vi "Change Settings.vi"(8 "error in (no error)":errorcluster) -> (0 "error out":errorcluster)   [LabVIEW 2020, in "MacroAssert.lvlib"]
doc: "Displays a window to change any settings that have been established in the application."
uses:
  MacroAssert.lvlib
  CTLs/Hotkey Type.ctl
  CTLs/Hotkey Values.ctl
  CTLs/FGV Actions.ctl
  2b057859-5186-41e9-9ab4-790756e7a186.vi
  a5ac09e5-38d3-43bc-9feb-68748838b8f7.vi
  <vilib>/Utility/inputDevices.llb/closeKeyboard.vi
  <vilib>/Utility/inputDevices.llb/keyboardAcquire.vi
  FaKI State Machine/FaKI State Machine.lvlib
panel:
  in  "Hotkey Type":T1
  in  "Start/Stop":bool
  in  "Exit":bool
  # "Change Hotkey\nPress Start Listening and hold down a key combination for five seconds to assign it as a hotkey."
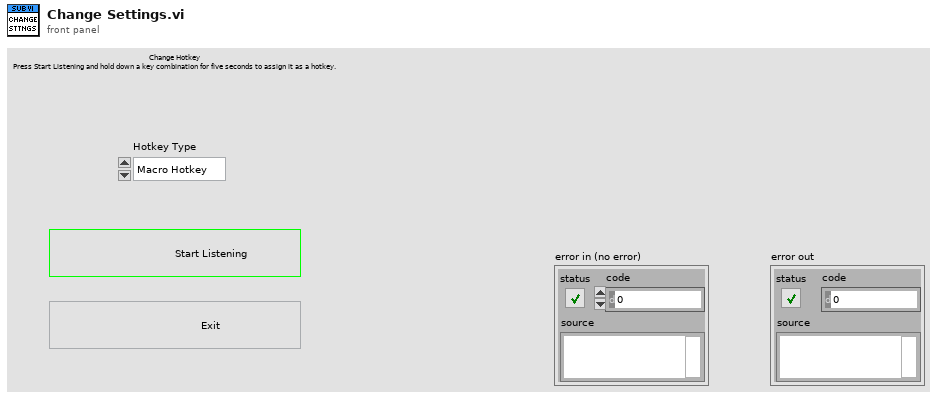
[diagram p1: front panel]
types:
  T1 = typedef "MacroAssert.lvlib/Hotkey Type.ctl" = enum16{"Macro Hotkey", "Abort Hotkey"}
  T2 = enum32{"Invalid", "Standard", "Closed", "Hidden", "Minimized", "Maximized"}
  T3 = enum32{"invalid app kind", "Development System", "Run Time System", "Student Edition", "Embedded LabVIEW", "Evaluation", "Custom"}
  T4 = typedef "MacroAssert.lvlib/FGV Actions.ctl" = enum16{"Read", "Write"}
  T5 = typedef "MacroAssert.lvlib/Hotkey Values.ctl" = cluster{"Macro Hotkey":enum16{"0", "1", "2", "3", "4", "5", "6", "7", "8", "9", "A", "B", "C", "D", "E", "F", "G", "H", "I", "J", "K", "L", "M", "N", "O", "P", "Q", "R", "S", "T", "U", "V", "W", "X", "Y", "Z", "F1", "F2", "F3", "F4", "F5", "F6", "F7", "F8", "F9", "F10", "F11", "F12", "F13", "F14", "F15", "ADD", "BACK", "BACKSLASH", "CAPITAL", "COMMA", "DECIMAL", "DELETE", "DIVIDE", "DOWN", "END", "EQUALS", "ESCAPE", "GRAVE (`)", "HOME", "INSERT", "LBRACKET", "LCONTROL", "LEFT", "L ALT", "LSHIFT", "LWIN", "MINUS", "MULTIPLY", "NEXT", "NUMLOCK", "NUMPAD_0", "NUMPAD_1", "NUMPAD_2", "NUMPAD_3", "NUMPAD_4", "NUMPAD_5", "NUMPAD_6", "NUMPAD_7", "NUMPAD_8", "NUMPAD_9", "PAUSE", "PERIOD", "PRIOR (PG UP)", "RBRACKET", "RCONTROL", "RETURN", "RIGHT", "R ALT", "RSHIFT", "RWIN", "SCROLL", "SEMICOLON", "SLASH", "SPACE", "SUBTRACT", "TAB", "UP", "ENTER (num pad)", "' (quote)"}[], "Abort Hotkey":enum16{"0", "1", "2", "3", "4", "5", "6", "7", "8", "9", "A", "B", "C", "D", "E", "F", "G", "H", "I", "J", "K", "L", "M", "N", "O", "P", "Q", "R", "S", "T", "U", "V", "W", "X", "Y", "Z", "F1", "F2", "F3", "F4", "F5", "F6", "F7", "F8", "F9", "F10", "F11", "F12", "F13", "F14", "F15", "ADD", "BACK", "BACKSLASH", "CAPITAL", "COMMA", "DECIMAL", "DELETE", "DIVIDE", "DOWN", "END", "EQUALS", "ESCAPE", "GRAVE (`)", "HOME", "INSERT", "LBRACKET", "LCONTROL", "LEFT", "L ALT", "LSHIFT", "LWIN", "MINUS", "MULTIPLY", "NEXT", "NUMLOCK", "NUMPAD_0", "NUMPAD_1", "NUMPAD_2", "NUMPAD_3", "NUMPAD_4", "NUMPAD_5", "NUMPAD_6", "NUMPAD_7", "NUMPAD_8", "NUMPAD_9", "PAUSE", "PERIOD", "PRIOR (PG UP)", "RBRACKET", "RCONTROL", "RETURN", "RIGHT", "R ALT", "RSHIFT", "RWIN", "SCROLL", "SEMICOLON", "SLASH", "SPACE", "SUBTRACT", "TAB", "UP", "ENTER (num pad)", "' (quote)"}[]}
  T6 = cluster{"Core":cluster{"Current VI Reference":refnum<vi>, "Close Panel on Exit?":bool}, "Keyboard":refnum<k1>, "Last":enum16{"0", "1", "2", "3", "4", "5", "6", "7", "8", "9", "A", "B", "C", "D", "E", "F", "G", "H", "I", "J", "K", "L", "M", "N", "O", "P", "Q", "R", "S", "T", "U", "V", "W", "X", "Y", "Z", "F1", "F2", "F3", "F4", "F5", "F6", "F7", "F8", "F9", "F10", "F11", "F12", "F13", "F14", "F15", "ADD", "BACK", "BACKSLASH", "CAPITAL", "COMMA", "DECIMAL", "DELETE", "DIVIDE", "DOWN", "END", "EQUALS", "ESCAPE", "GRAVE (`)", "HOME", "INSERT", "LBRACKET", "LCONTROL", "LEFT", "L ALT", "LSHIFT", "LWIN", "MINUS", "MULTIPLY", "NEXT", "NUMLOCK", "NUMPAD_0", "NUMPAD_1", "NUMPAD_2", "NUMPAD_3", "NUMPAD_4", "NUMPAD_5", "NUMPAD_6", "NUMPAD_7", "NUMPAD_8", "NUMPAD_9", "PAUSE", "PERIOD", "PRIOR (PG UP)", "RBRACKET", "RCONTROL", "RETURN", "RIGHT", "R ALT", "RSHIFT", "RWIN", "SCROLL", "SEMICOLON", "SLASH", "SPACE", "SUBTRACT", "TAB", "UP", "ENTER (num pad)", "' (quote)"}[], "Hotkeys":T5}
  T7 = enum16{"0", "1", "2", "3", "4", "5", "6", "7", "8", "9", "A", "B", "C", "D", "E", "F", "G", "H", "I", "J", "K", "L", "M", "N", "O", "P", "Q", "R", "S", "T", "U", "V", "W", "X", "Y", "Z", "F1", "F2", "F3", "F4", "F5", "F6", "F7", "F8", "F9", "F10", "F11", "F12", "F13", "F14", "F15", "ADD", "BACK", "BACKSLASH", "CAPITAL", "COMMA", "DECIMAL", "DELETE", "DIVIDE", "DOWN", "END", "EQUALS", "ESCAPE", "GRAVE (`)", "HOME", "INSERT", "LBRACKET", "LCONTROL", "LEFT", "L ALT", "LSHIFT", "LWIN", "MINUS", "MULTIPLY", "NEXT", "NUMLOCK", "NUMPAD_0", "NUMPAD_1", "NUMPAD_2", "NUMPAD_3", "NUMPAD_4", "NUMPAD_5", "NUMPAD_6", "NUMPAD_7", "NUMPAD_8", "NUMPAD_9", "PAUSE", "PERIOD", "PRIOR (PG UP)", "RBRACKET", "RCONTROL", "RETURN", "RIGHT", "R ALT", "RSHIFT", "RWIN", "SCROLL", "SEMICOLON", "SLASH", "SPACE", "SUBTRACT", "TAB", "UP", "ENTER (num pad)", "' (quote)"}[]
  T8 = cluster{"Current VI Reference":refnum<vi>, "Close Panel on Exit?":bool}
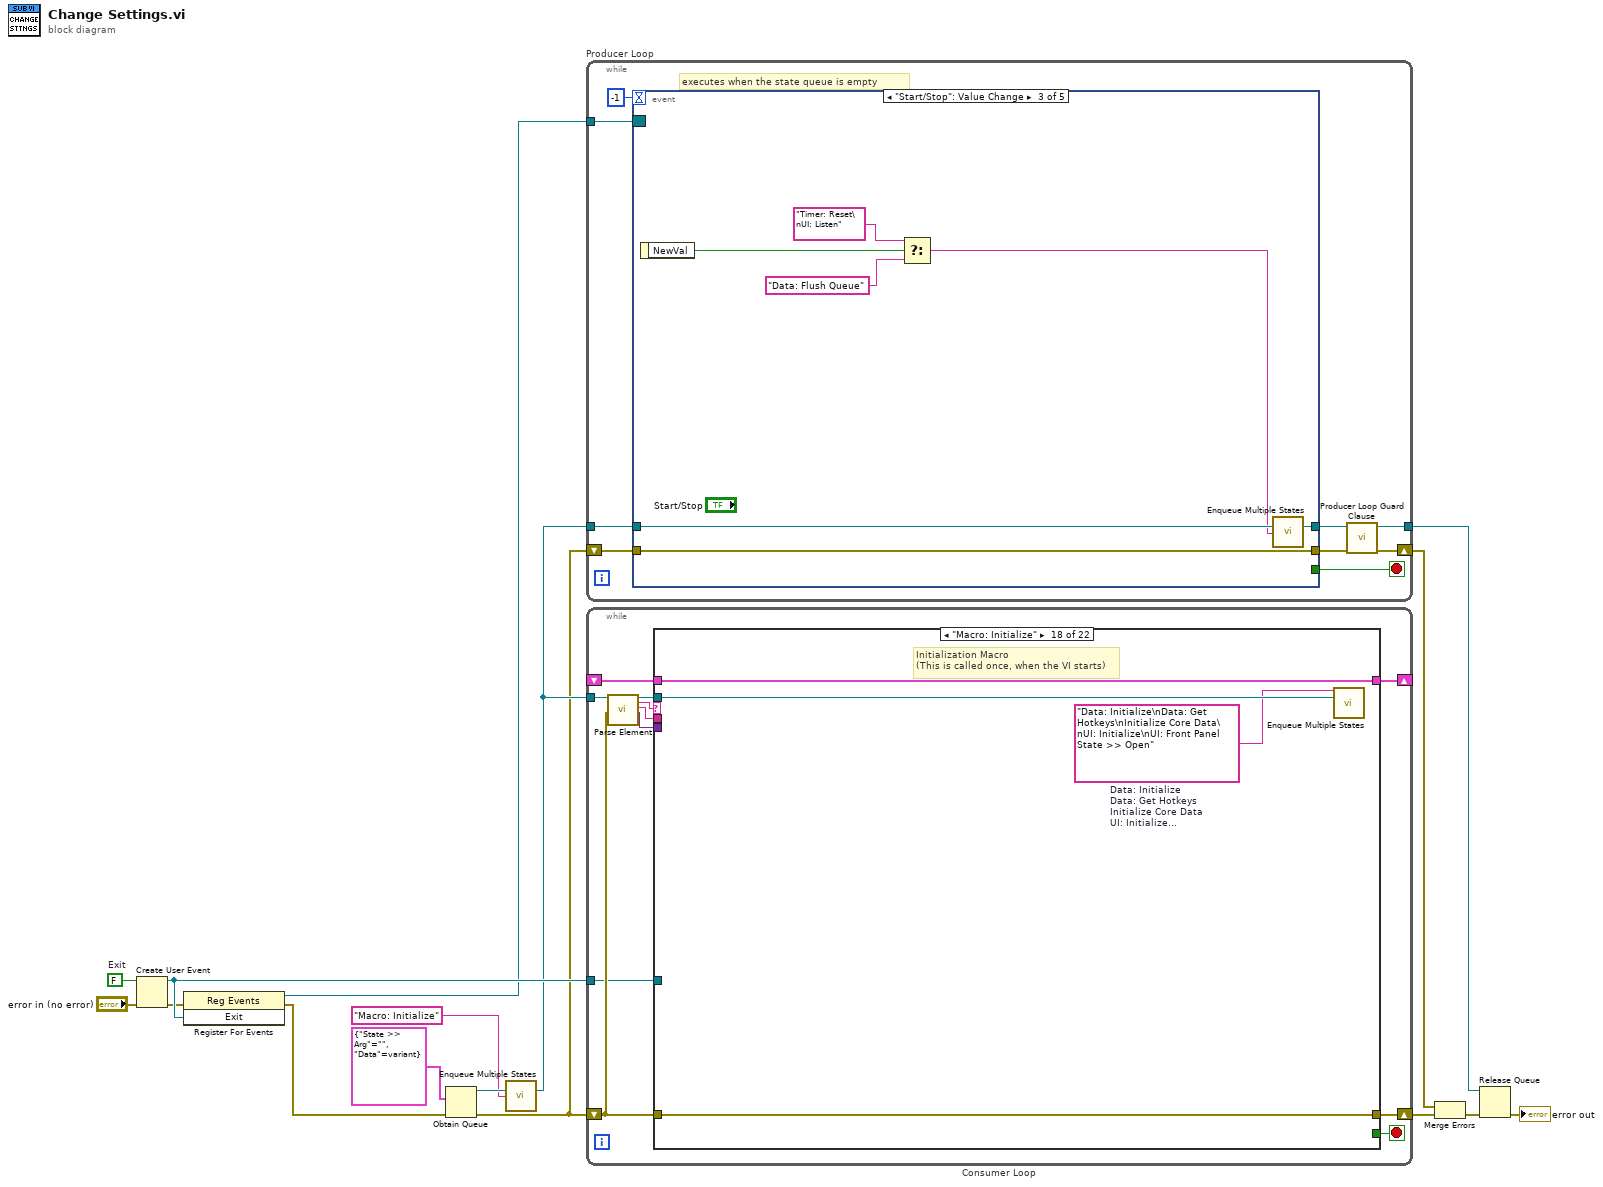
[diagram p0: block diagram]
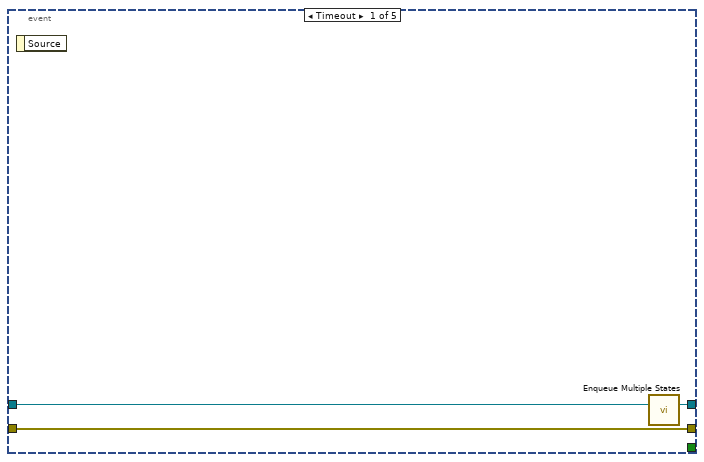
[diagram p2: hidden frame]
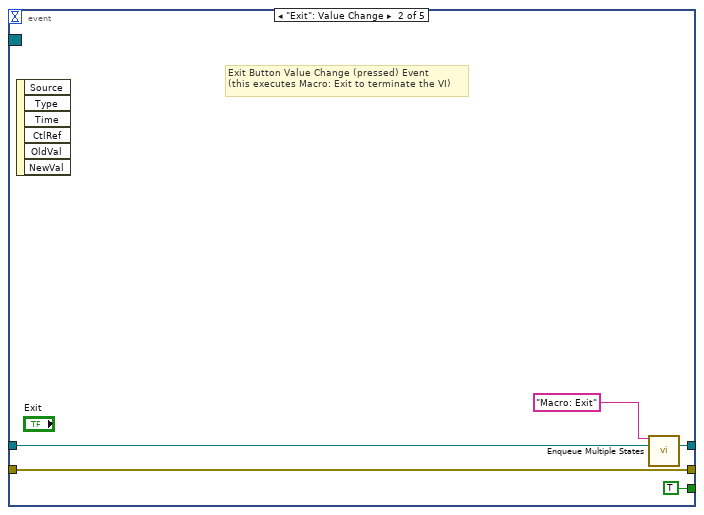
[diagram p3: hidden frame]
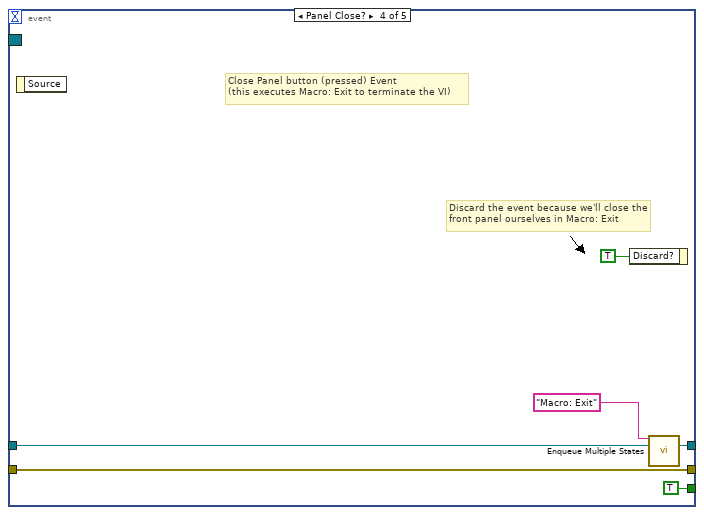
[diagram p4: hidden frame]
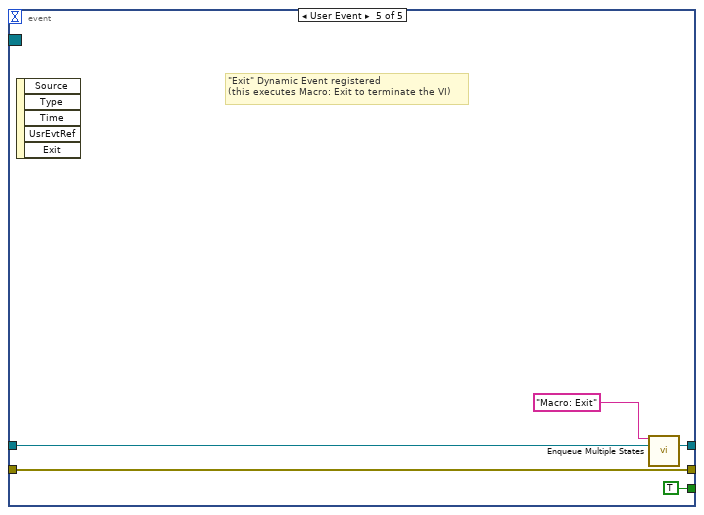
[diagram p5: hidden frame]
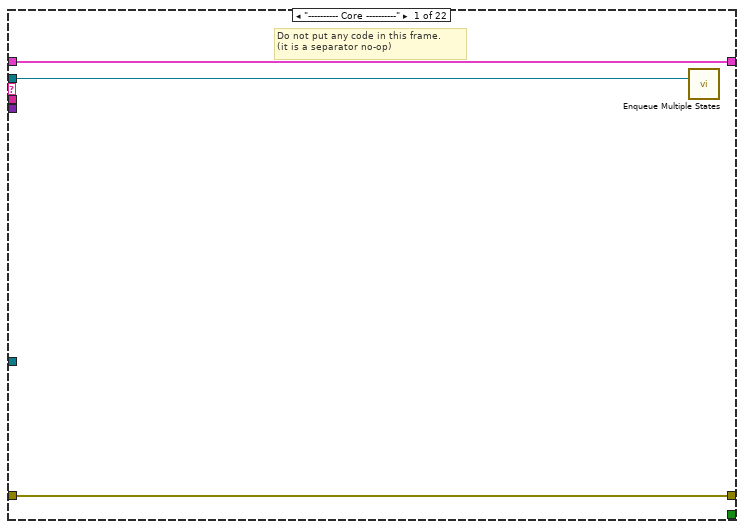
[diagram p6: hidden frame]
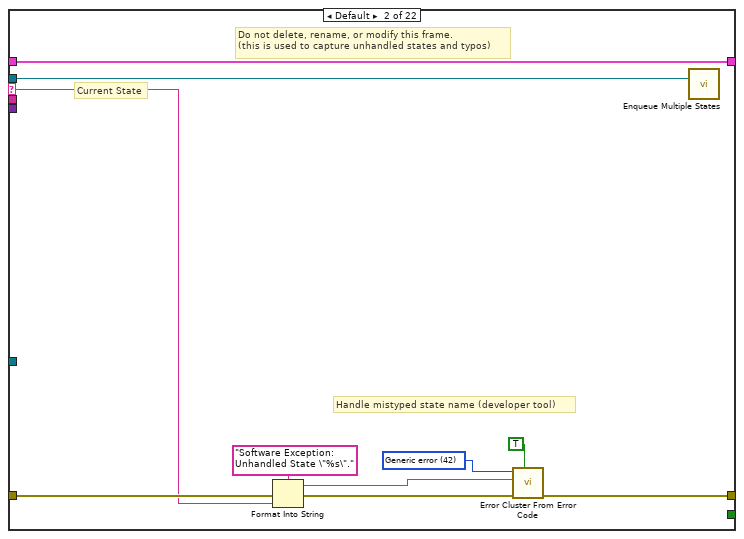
[diagram p7: hidden frame]
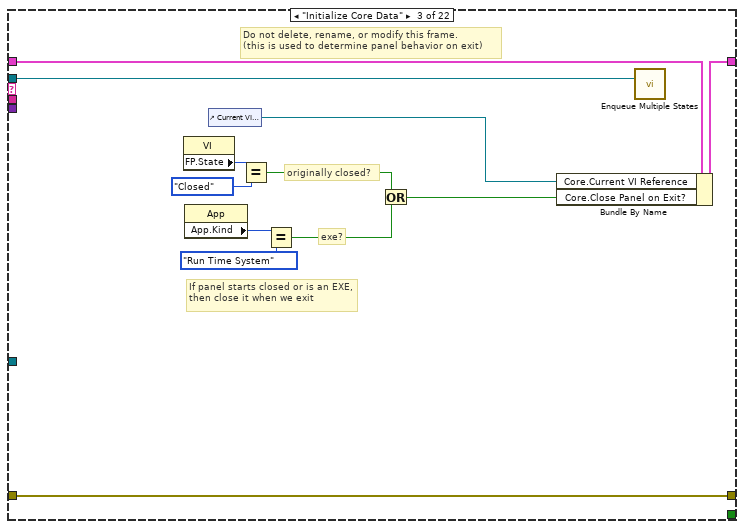
[diagram p8: hidden frame]
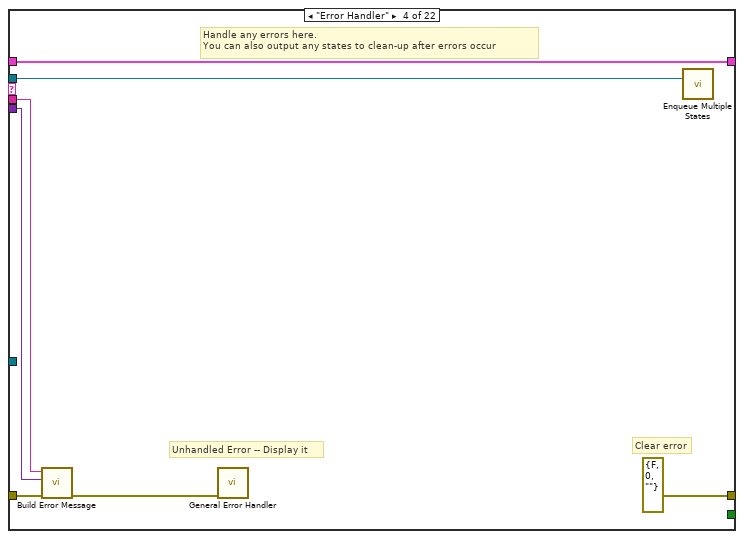
[diagram p9: hidden frame]
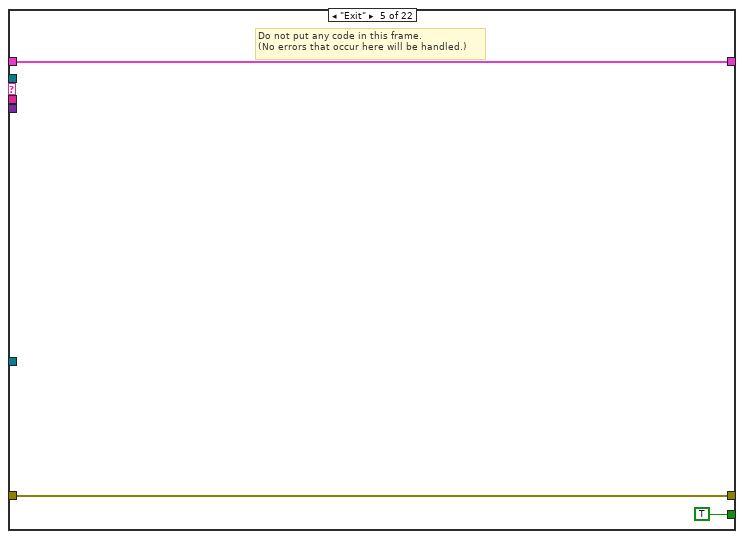
[diagram p10: hidden frame]
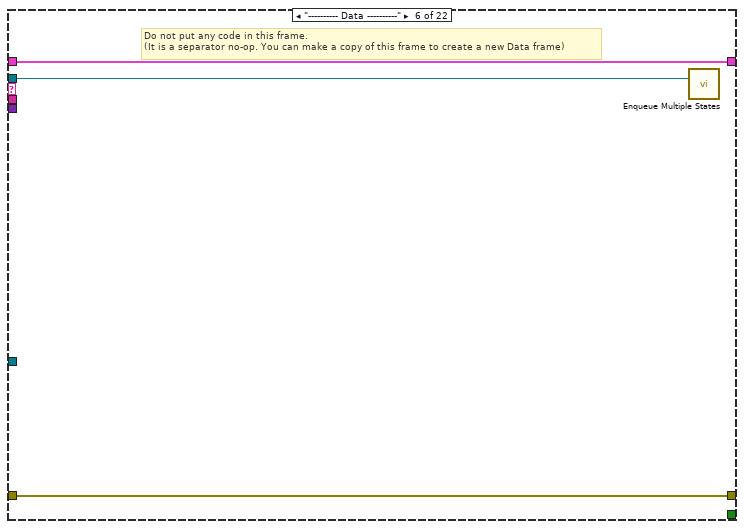
[diagram p11: hidden frame]
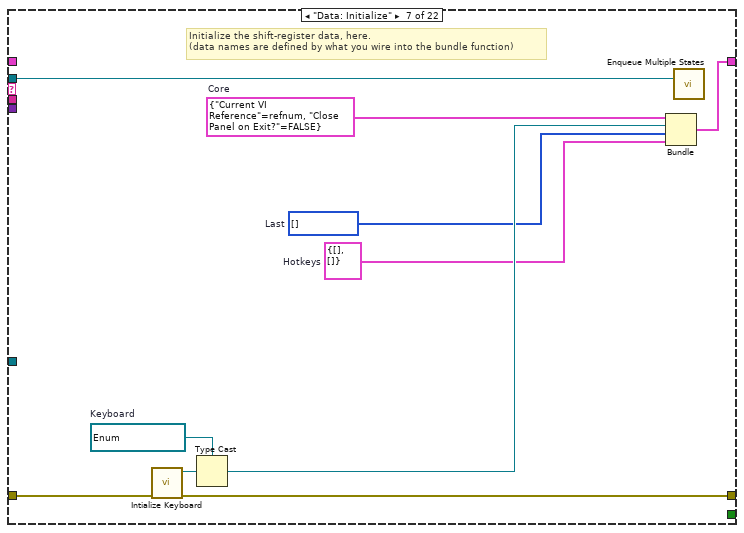
[diagram p12: hidden frame]
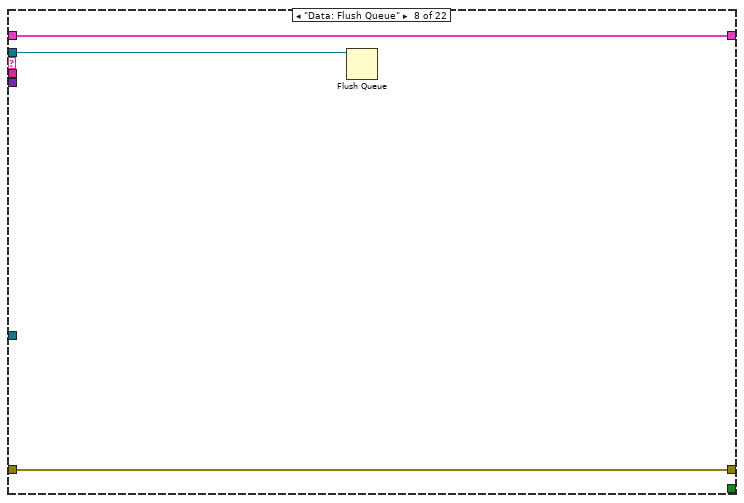
[diagram p13: hidden frame]
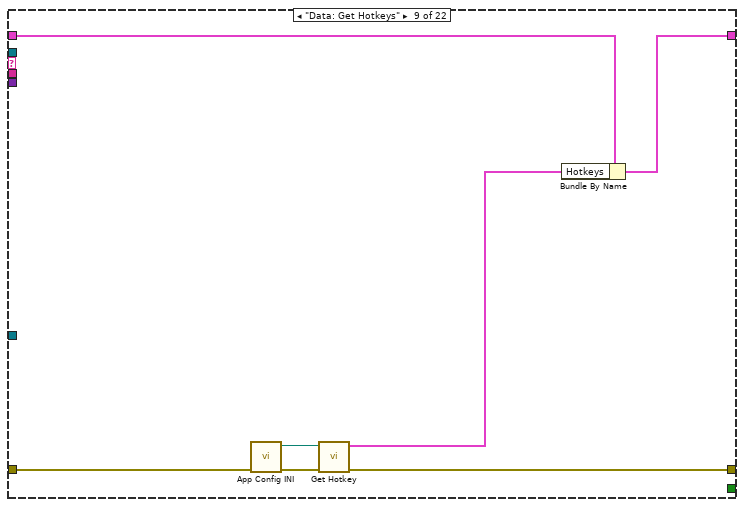
[diagram p14: hidden frame]
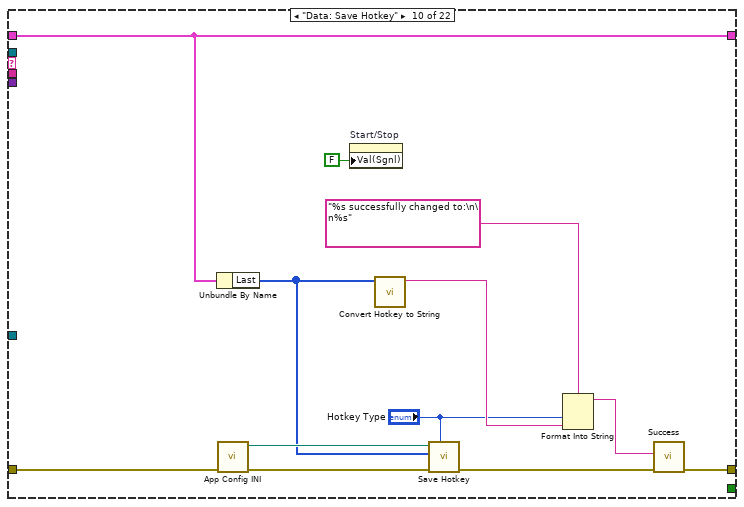
[diagram p15: hidden frame]
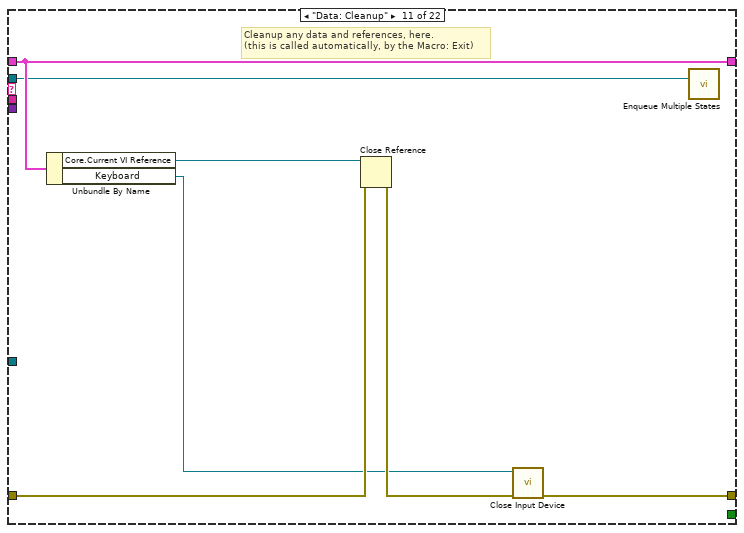
[diagram p16: hidden frame]
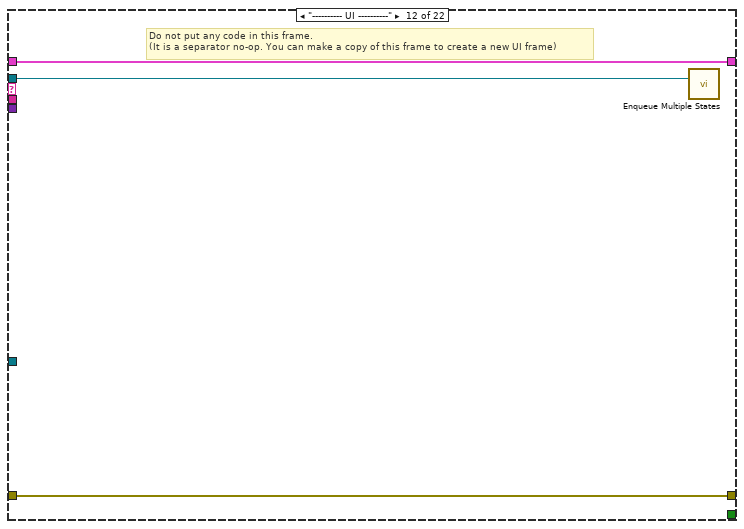
[diagram p17: hidden frame]
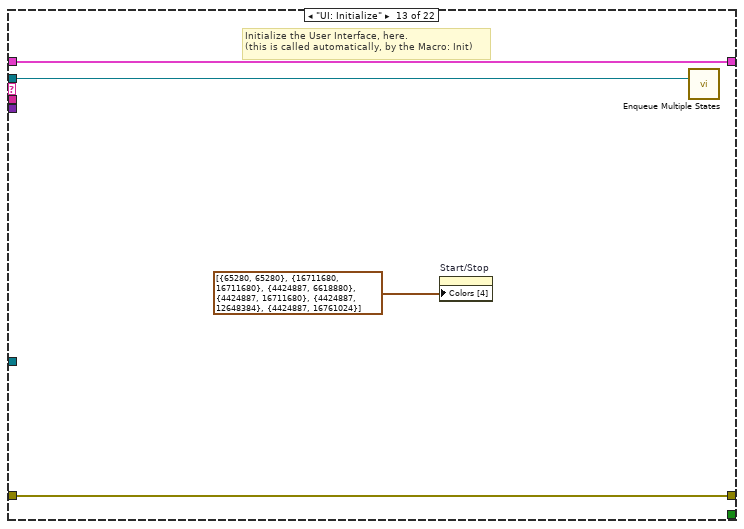
[diagram p18: hidden frame]
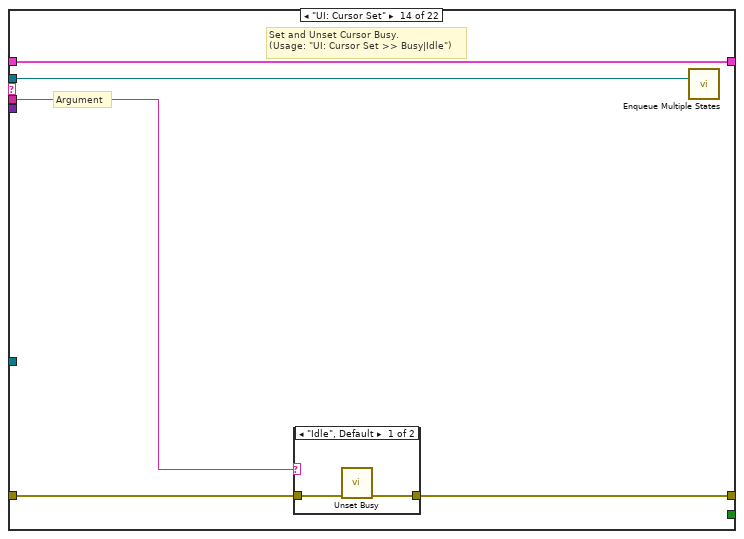
[diagram p19: hidden frame]
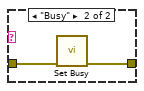
[diagram p20: hidden frame]
diagram:
  w13 = FALSE  # Exit
  n1 = Create User Event(user event datatype=w13, error in="error in (no error)") -> (user event=w16:refnum<user-event>, error out=w12:errorcluster)
  n2 = register-events(error in=w12, w16) -> (reference out=w15:refnum<event-registration>, error out=w14:errorcluster)  [unwired: 1 in]
  n3 = Obtain Queue(element data type=cluster{"State >> Arg":string, "Data":variant} {"State >> Arg"="", "Data"=variant}, error in (no error)=w14) -> (queue out=w6:refnum<queue>, error out=w3:errorcluster)  [unwired: 3 in, 1 out]
  n4 = call "Enqueue Multiple States.vi"("queue in"=w6, "State(s) at Back"="Macro: Initialize") -> ("queue out"=w7:refnum<queue>)  [unwired: 13 in]
  n5 = while "Producer Loop" {
    shift-right: [w20] -> w9
    shift-left: w3 -> [w25]
    tunnel: w15 -> [w17]
    tunnel: w7 -> [w23]
    tunnel: [w18] -> w11
    stop <- w22 stop-if-true
    # "executes when the state queue is empty"
    n6 = event shown="[2] \"Start/Stop\": Value Change" {
      selector: w17 -> [_ _ _ _ _]
      dyn-events: _ -> [_ _ _ _ _]
      timeout: -1 ("Timeout") -> [_ _ _ _ _]
      tunnel: [w26 w33 w40 w46 w51] -> w21
      tunnel: w25 -> [w26 w33 w40 w46 w51]
      tunnel: w23 -> [w27 w32 w39 w43 w49]
      tunnel: [w28 w30 w38 w42 w48] -> w19
      tunnel: [_ TRUE _ TRUE TRUE] -> w22
      event Timeout {
        n7 = event-data() -> ()  [unwired: 1 in, 1 out]
        n8 = call "Enqueue Multiple States.vi"("queue in"=w27) -> ("queue out"=w28:refnum<queue>)  [unwired: 14 in]
      }
      event "Exit": Value Change {
        # "Exit Button Value Change (pressed) Event\n(this executes Macro: Exit to terminate the VI)"
        n9 = event-data() -> ()  [unwired: 1 in, 6 out]
        n10 = call "Enqueue Multiple States.vi"("State(s) at Front"="Macro: Exit", "queue in"=w32) -> ("queue out"=w30:refnum<queue>)  [unwired: 13 in]
      }
      event "Start/Stop": Value Change {
        n11 = event-data() -> ("NewVal"=w37:bool)  [unwired: 1 in]
        n12 = Select(t="Timer: Reset\nUI: Listen", s=w37, f="Data: Flush Queue") -> (s? t:f=w34:string)
        n13 = call "Enqueue Multiple States.vi"("queue in"=w39, "State(s) at Back"=w34) -> ("queue out"=w38:refnum<queue>)  [unwired: 13 in]
      }
      event Panel Close? {
        # "Discard the event because we'll close the front panel ourselves in Macro: Exit"
        # "Close Panel button (pressed) Event\n(this executes Macro: Exit to terminate the VI)"
        n14 = event-data() -> ()  [unwired: 1 in, 1 out]
        n15 = event-data("Discard?"=TRUE) -> ()  [unwired: 1 in, 1 out]
        n16 = call "Enqueue Multiple States.vi"("State(s) at Front"="Macro: Exit", "queue in"=w43) -> ("queue out"=w42:refnum<queue>)  [unwired: 13 in]
      }
      event User Event {
        # "\"Exit\" Dynamic Event registered\n(this executes Macro: Exit to terminate the VI)"
        n17 = event-data() -> ()  [unwired: 1 in, 5 out]
        n18 = call "Enqueue Multiple States.vi"("State(s) at Front"="Macro: Exit", "queue in"=w49) -> ("queue out"=w48:refnum<queue>)  [unwired: 13 in]
      }
    }
    n19 = call "Producer Loop Guard Clause.vi"("error in (no error)"=w21, "queue in"=w19) -> ("error out"=w20:errorcluster, "queue out"=w18:refnum<queue>)  [unwired: 8 in]
  }
  n20 = while "Consumer Loop" {
    shift-right: [w59] -> _
    shift-left: _ -> [w58]
    shift-right: [w62] -> w8
    shift-left: w3 -> [w61]
    tunnel: w7 -> [w57]
    tunnel: w16 -> [w52]
    stop <- w60 stop-if-true
    n21 = call "Parse Element.vi"("queue in"=w57, "error in (no error)"=w61) -> ("queue out"=w56:refnum<queue>, "State"=w55:string, "Arg"=w54:string, "Data"=w53:variant)  [unwired: 14 in]
    n22 = case shown="\"Macro: Initialize\"" w55 {
      selector: w55 -> [_ w67 _ _ _ _ _ _ _ _ _ _ _ _ _ _ _ _ _ _ _ _]
      tunnel: w56 -> [w63 w66 w76 w92 _ w98 w108 w113 _ _ w136 w140 w144 w147 w156 w239 w262 w266 w272 w278 _ w287]
      tunnel: w54 -> [_ _ _ w88 _ _ _ _ _ _ _ _ _ w148 w157 _ _ _ _ _ _ _]
      tunnel: w58 -> [w64 w69 w82 w93 w96 w99 _ w112 w119 w125 w137 w141 w145 w149 w159 w238 w263 w267 w276 w279 w285 w294]
      tunnel: [w65 w74 w87 errorcluster {"status"=FALSE, "code"=0, "source"=""} ("error out") w97 w100 w103 w111 w117 w130 w134 w142 w146 w150 w160 w247 w264 w268 w277 w280 w283 w292] -> w62
      tunnel: w61 -> [w65 w73 w87 w91 w97 w100 w105 w111 w120 w128 w139 w142 w146 w151 w161 w248 w264 w268 w277 w280 w284 w293]
      tunnel: [_ _ _ _ TRUE _ _ _ _ _ _ _ _ _ _ _ _ _ _ _ _ _] -> w60
      tunnel: [w64 w69 w86 w93 w96 w99 w110 w112 w118 w125 w137 w141 w145 w149 w159 w237 w263 w267 w276 w279 w285 w294] -> w59
      tunnel: w53 -> [_ _ _ w89 _ _ _ _ _ _ _ _ _ _ _ _ _ _ _ _ _ _]
      tunnel: w52 -> [_ _ _ _ _ _ _ _ _ _ _ _ _ _ _ _ _ _ _ _ _ _]
      frame "---------- Core ----------" {
        # "Do not put any code in this frame.\n(it is a separator no-op)"
        n23 = call "Enqueue Multiple States.vi"("queue in"=w63) -> ()  [unwired: 14 in, 1 out]
      }
      frame Default {
        w71 = 42 items=["No error", "Argument error", "Memory is full", "Out of zone", "End of file", "File already open", "Generic file I/O error", "File not found", "File permission error", "Disk is full", "Duplicate path", "Too many files open", "System feature not enabled", "Resource file not found", "Cannot add resource", "Resource not found", "Image not found", "Image memory error", "Pen does not exist", "Config type invalid", "Config token not found", "Config parse error", "Config memory error", "Bad external code format", "Bad external code offset", "External code not present", "Null window", "Destroy window error", "Null menu", "Print aborted", "Bad print record", "Print driver error", "Windows error during printing", "Memory error during printing", "Print dialog error", "Generic print error", "Invalid device refnum", "Device not found", "Device parameter error", "Device unit error", "Cannot open device", "Device call aborted", "Generic error", "Cancelled by user", "Object ID too low", "Object ID too high", "Object not in heap", "Unknown heap", "Unknown object (invalid DefProc)", "Unknown object (DefProc not in table)", "Message out of range", "Invalid (null) method", "Unknown message", "Manager call not supported", "Bad address", "Network operation in progress", "Network operation timed out", "Connection is busy", "Network attribute not supported", "Network error", "Address in use", "System out of memory", "Connection aborted", "Connection refused", "Not connected", "Already connected", "Connection closed", "Initialization error (interapplication manager)", "Bad occurrence", "Wait on unbound occurrence handler", "Occurrence queue overflow", "Datalog type conflict", "Unused", "Unrecognized type (interapplication manager)", "Memory corrupt", "Failed to make temporary DLL", "Old CIN version", "Drag socket not found", "Failed to load drop-object", "Failed to register OLE object", "Failed to release OLE object", "Format specifier type mismatch", "Unknown format specifier", "Too few format specifiers", "Too many format specifiers", "Scan failed", "Newer CIN version", "Error converting to variant", "Runtime menu error", "Password tampered", "Variant attribute not found", "Incompatible variant data type", "Event data is not available", "Event Store is not present", "Occurrence is not found", "Event Queue is not created", "Event info is not available", "Refnum passed is NULL", "Error retrieving Class GUID", "Error retrieving CoClass GUID", "Error retrieving TypeLib GUID.", "Bad built application magic bytes.", "Specific driver is different from the specific driver associated with the Logical Name.", "There is no session opened to the class driver.", "Max Error", "MAX - Error with config objects", "MAX - Error loading configuration", "MAX - Group not supported"]
        # "Current State"
        # "Do not delete, rename, or modify this frame.\n(this is used to capture unhandled states and typos)"
        # "Handle mistyped state name (developer tool)"
        n24 = Format Into String(format string="Software Exception: Unhandled State \"%s\"." ("message"), error in=w73, w67) -> (resulting string=w70:string, error out=w75:errorcluster)  [unwired: 1 in]
        n25 = call <vilib>:"Error Cluster From Error Code.vi"("show call chain? (False)"=TRUE, "error in (no error)"=w75, "error message (\"\")"=w70, "error code (0)"=w71) -> ("error out"=w74:errorcluster)  [unwired: 5 in]
        n26 = call "Enqueue Multiple States.vi"("queue in"=w66) -> ()  [unwired: 14 in, 1 out]
      }
      frame "Initialize Core Data" {
        # "Do not delete, rename, or modify this frame.\n(this is used to determine panel behavior on exit)"
        # "originally closed?"
        # "exe?"
        # "If panel starts closed or is an EXE, then close it when we exit"
        n27 = property class="VI"() -> ("FP.State"=w79:T2)  [unwired: 2 in, 2 out]
        n28 = property class="App"() -> ("App.Kind"=w85:T3)  [unwired: 2 in, 2 out]
        n29 = control-ref of="Current VI Reference"() -> (w80:refnum<vi>)
        n30 = Equal?(x=w79, y=T2."Closed" ("Front Panel Window:State")) -> (x = y?=w77:bool)
        n31 = Equal?(x=w85, y=T3."Run Time System" ("Application:Kind")) -> (x = y?=w83:bool)
        n32 = Or(x=w77, y=w83) -> (x .or. y?=w81:bool)
        n33 = Bundle By Name(cluster=w82, "Core.Current VI Reference"=w80, "Core.Close Panel on Exit?"=w81) -> (w86:T6)
        n34 = call "Enqueue Multiple States.vi"("queue in"=w76) -> ()  [unwired: 14 in, 1 out]
      }
      frame "Error Handler" {
        # "Unhandled Error -- Display it"
        # "Handle any errors here.\nYou can also output any states to clean-up after errors occur"
        # "Clear error"
        n35 = call "Build Error Message.vi"("error in (no error)"=w91, "Data"=w89, "Arg"=w88) -> ("error out"=w90:errorcluster)  [unwired: 8 in]
        n36 = call <vilib>:"General Error Handler.vi"("error in (no error)"=w90) -> ()  [unwired: 10 in, 5 out]
        n37 = call "Enqueue Multiple States.vi"("queue in"=w92) -> ()  [unwired: 14 in, 1 out]
      }
      frame "Exit" {
        # "Do not put any code in this frame.\n(No errors that occur here will be handled.)"
      }
      frame "---------- Data ----------" {
        # "Do not put any code in this frame.\n(It is a separator no-op. You can make a copy of this frame to create a new Data frame)"
        n38 = call "Enqueue Multiple States.vi"("queue in"=w98) -> ()  [unwired: 14 in, 1 out]
      }
      frame "Data: Initialize" {
        w101 = T5 {"Macro Hotkey"=[], "Abort Hotkey"=[]}  # Hotkeys
        w102 = T7 [] items=["0", "1", "2", "3", "4", "5", "6", "7", "8", "9", "A", "B", "C", "D", "E", "F", "G", "H", "I", "J", "K", "L", "M", "N", "O", "P", "Q", "R", "S", "T", "U", "V", "W", "X", "Y", "Z", "F1", "F2", "F3", "F4", "F5", "F6", "F7", "F8", "F9", "F10", "F11", "F12", "F13", "F14", "F15", "ADD", "BACK", "BACKSLASH", "CAPITAL", "COMMA", "DECIMAL", "DELETE", "DIVIDE", "DOWN", "END", "EQUALS", "ESCAPE", "GRAVE (`)", "HOME", "INSERT", "LBRACKET", "LCONTROL", "LEFT", "L ALT", "LSHIFT", "LWIN", "MINUS", "MULTIPLY", "NEXT", "NUMLOCK", "NUMPAD_0", "NUMPAD_1", "NUMPAD_2", "NUMPAD_3", "NUMPAD_4", "NUMPAD_5", "NUMPAD_6", "NUMPAD_7", "NUMPAD_8", "NUMPAD_9", "PAUSE", "PERIOD", "PRIOR (PG UP)", "RBRACKET", "RCONTROL", "RETURN", "RIGHT", "R ALT", "RSHIFT", "RWIN", "SCROLL", "SEMICOLON", "SLASH", "SPACE", "SUBTRACT", "TAB", "UP", "ENTER (num pad)", "' (quote)"]  # Last
        w106 = refnum<k1> refnum items=["KEYBOARD"]  # Keyboard
        w109 = T8 {"Current VI Reference"=refnum, "Close Panel on Exit?"=FALSE}  # Core
        # "Initialize the shift-register data, here.\n(data names are defined by what you wire into the bundle function)"
        n39 = call <vilib>:"Intialize Keyboard.vi"("error in (no error)"=w105) -> ("error out"=w103:errorcluster, "device ID"=w107:refnum<k1>)  [unwired: 9 in]
        n40 = Type Cast(type=w106, x=w107) -> (*(type *) &x=w104:refnum<k1>)
        n41 = Bundle("Core"=w109, "Keyboard"=w104, "Last"=w102, "Hotkeys"=w101) -> (w110:T6)  [unwired: 1 in]
        n42 = call "Enqueue Multiple States.vi"("queue in"=w108) -> ()  [unwired: 14 in, 1 out]
      }
      frame "Data: Flush Queue" {
        n43 = Flush Queue(queue=w113) -> ()  [unwired: 1 in, 3 out]
      }
      frame "Data: Get Hotkeys" {
        n44 = call "App Config INI.vi"("error in (no error)"=w120) -> ("error out"=w115:errorcluster, "App Config"=w114:path)  [unwired: 9 in]
        n45 = call "Get Hotkey.vi"("error in (no error)"=w115, "File Path"=w114) -> ("error out"=w117:errorcluster, "Hotkey Values"=w116:T5)  [unwired: 8 in]
        n46 = Bundle By Name(cluster=w119, "Hotkeys"=w116) -> (w118:T6)
      }
      frame "Data: Save Hotkey" {
        n47 = Unbundle By Name(w125) -> ("Last"=w122:T7)
        n48 = call "App Config INI.vi"("error in (no error)"=w128) -> ("error out"=w124:errorcluster, "App Config"=w123:path)  [unwired: 9 in]
        n49 = property on="Start/Stop" class="Bool (strict)"("Val(Sgnl)"=FALSE ("Value (Signaling)")) -> ()  [unwired: 2 in, 2 out]
        n50 = call "Convert Hotkey to String.vi"("Hotkey"=w122) -> ("String"=w126:string)  [unwired: 10 in]
        n51 = call "Save Hotkey.vi"("Hotkey Type"="Hotkey Type", "error in (no error)"=w124, "Hotkey"=w122, "File Path"=w123) -> ("error out"=w127:errorcluster)  [unwired: 7 in]
        n52 = Format Into String(format string="%s successfully changed to:\n\n%s", "Hotkey Type", w126) -> (resulting string=w131:string)  [unwired: 2 in, 1 out]
        n53 = call "Success"("error in (no error)"=w127, "Message"=w131) -> ("error out"=w130:errorcluster)  [unwired: 8 in, 1 out]
      }
      frame "Data: Cleanup" {
        # "Cleanup any data and references, here.\n(this is called automatically, by the Macro: Exit)"
        n54 = Unbundle By Name(w137) -> ("Core.Current VI Reference"=w138:refnum<vi>, "Keyboard"=w133:refnum<k1>)
        n55 = Close Reference(reference=w138, error in (no error)=w139) -> (error out=w135:errorcluster)
        n56 = call-poly <vilib>:"Close Input Device.vi"("error in (no error)"=w135, "device ID"=w133) -> ("error out"=w134:errorcluster)  [unwired: 8 in]
        n57 = call "Enqueue Multiple States.vi"("queue in"=w136) -> ()  [unwired: 14 in, 1 out]
      }
      frame "---------- UI ----------" {
        # "Do not put any code in this frame.\n(It is a separator no-op. You can make a copy of this frame to create a new UI frame)"
        n58 = call "Enqueue Multiple States.vi"("queue in"=w140) -> ()  [unwired: 14 in, 1 out]
      }
      frame "UI: Initialize" {
        # "Initialize the User Interface, here.\n(this is called automatically, by the Macro: Init)"
        n59 = property on="Start/Stop" class="Bool (strict)"("Colors [4]"=cluster{u32, u32}[] [{65280, 65280}, {16711680, 16711680}, {4424887, 6618880}, {4424887, 16711680}, {4424887, 12648384}, {4424887, 16761024}]) -> ()  [unwired: 2 in, 2 out]
        n60 = call "Enqueue Multiple States.vi"("queue in"=w144) -> ()  [unwired: 14 in, 1 out]
      }
      frame "UI: Cursor Set" {
        # "Argument"
        # "Set and Unset Cursor Busy.\n(Usage: \"UI: Cursor Set >> Busy|Idle\")"
        n61 = case shown="\"Idle\", Default" w148 {
          tunnel: w151 -> [w153 w155]
          tunnel: [w152 w154] -> w150
          frame "Idle", Default {
            n62 = call <vilib>:"Unset Busy.vi"("error in (no error)"=w153) -> ("error out"=w152:errorcluster)  [unwired: 10 in]
          }
          frame "Busy" {
            n63 = call <vilib>:"Set Busy.vi"("error in (no error)"=w155) -> ("error out"=w154:errorcluster)  [unwired: 9 in, 1 out]
          }
        }
        n64 = call "Enqueue Multiple States.vi"("queue in"=w147) -> ()  [unwired: 14 in, 1 out]
      }
      frame "UI: Front Panel State" {
        # "Argument"
        # "Set Front Panel Open or Closed\n(Usage: \"UI: Front Panel State >> Open|Close\")"
        n65 = Unbundle By Name(w159) -> ("Core.Current VI Reference"=w158:refnum<vi>)
        n66 = case shown="\"Open\", \"Standard\", Default" w157 {
          tunnel: w161 -> [w168 w182 w194 w207 w220]
          tunnel: [w169 w183 w195 w208 w221] -> w160
          tunnel: w158 -> [w166 w180 w192 w205 w218]
          frame "Open", "Standard", Default {
            w162 = T2."Standard" ("State")
            n67 = property class="VI"(reference=w166, error in=w168) -> (reference out=w165:refnum<vi>, error out=w167:errorcluster, "FP.State"=w164:T2)
            n68 = Not Equal?(x=w164, y=w162) -> (x != y?=w163:bool)
            n69 = case shown="True" w163 {
              tunnel: [w174 w175] -> w169
              tunnel: w167 -> [w173 w175]
              tunnel: w165 -> [w171 _]
              tunnel: w162 -> [w170 _]
              frame True {
                n70 = invoke class="VI" method="FP.Open"(reference=w171, error in=w173, "Activate"=TRUE, "State"=w170) -> (error out=w174:errorcluster)  [unwired: 1 in, 4 out]
              }
              frame False {
              }
            }
          }
          frame "Close", "Closed" {
            n71 = property class="VI"(reference=w180, error in=w182) -> (reference out=w179:refnum<vi>, error out=w181:errorcluster, "FP.State"=w177:T2)
            n72 = Not Equal?(x=w177, y=T2."Closed" ("Front Panel Window:State")) -> (x != y?=w176:bool)
            n73 = case shown="True" w176 {
              tunnel: [w184 w187] -> w183
              tunnel: w181 -> [w184 w186]
              tunnel: w179 -> [_ w185]
              frame False {
              }
              frame True {
                n74 = invoke class="VI" method="FP.Close"(reference=w185, error in=w186) -> (error out=w187:errorcluster)  [unwired: 1 in, 2 out]
              }
            }
          }
          frame "Hidden", "Hide" {
            w188 = T2."Hidden" ("State")
            n75 = property class="VI"(reference=w192, error in=w194) -> (reference out=w191:refnum<vi>, error out=w193:errorcluster, "FP.State"=w190:T2)
            n76 = Not Equal?(x=w190, y=w188) -> (x != y?=w189:bool)
            n77 = case shown="True" w189 {
              tunnel: [w199 w200] -> w195
              tunnel: w193 -> [w198 w200]
              tunnel: w191 -> [w197 _]
              tunnel: w188 -> [w196 _]
              frame True {
                n78 = invoke class="VI" method="FP.Open"(reference=w197, error in=w198, "State"=w196) -> (error out=w199:errorcluster)  [unwired: 2 in, 4 out]
              }
              frame False {
              }
            }
          }
          frame "Minimize", "Minimized" {
            w201 = T2."Minimized" ("State")
            n79 = property class="VI"(reference=w205, error in=w207) -> (reference out=w204:refnum<vi>, error out=w206:errorcluster, "FP.State"=w203:T2)
            n80 = Not Equal?(x=w203, y=w201) -> (x != y?=w202:bool)
            n81 = case shown="True" w202 {
              tunnel: [w212 w213] -> w208
              tunnel: w206 -> [w211 w213]
              tunnel: w204 -> [w210 _]
              tunnel: w201 -> [w209 _]
              frame True {
                n82 = invoke class="VI" method="FP.Open"(reference=w210, error in=w211, "State"=w209) -> (error out=w212:errorcluster)  [unwired: 2 in, 4 out]
              }
              frame False {
              }
            }
          }
          frame "Maximize", "Maximized" {
            w214 = T2."Maximized" ("State")
            n83 = property class="VI"(reference=w218, error in=w220) -> (reference out=w217:refnum<vi>, error out=w219:errorcluster, "FP.State"=w216:T2)
            n84 = Not Equal?(x=w216, y=w214) -> (x != y?=w215:bool)
            n85 = case shown="True" w215 {
              tunnel: [w225 w226] -> w221
              tunnel: w219 -> [w224 w226]
              tunnel: w217 -> [w223 _]
              tunnel: w214 -> [w222 _]
              frame True {
                n86 = invoke class="VI" method="FP.Open"(reference=w223, error in=w224, "State"=w222) -> (error out=w225:errorcluster)  [unwired: 2 in, 4 out]
              }
              frame False {
              }
            }
          }
        }
        n87 = call "Enqueue Multiple States.vi"("queue in"=w156) -> ()  [unwired: 14 in, 1 out]
      }
      frame "UI: Listen" {
        n88 = Unbundle By Name(w238) -> ("Hotkeys"=w233:T5, "Last"=w245:T7, "Keyboard"=w252:refnum<k1>)
        n89 = call "Stall Data Flow.vim"("value in"=w252, "milliseconds to wait"=u32 1) -> ("value out"=w250:refnum<k1>)  [unwired: 1 out]
        n90 = Empty Array?(array=w245) -> (empty?=w246:bool)
        n91 = call-poly <vilib>:"Acquire Input Data.vi"("device ID"=w250, "error in (no error)"=w248) -> ("keys pressed"=w251:T7, "error out"=w247:errorcluster)  [unwired: 15 in, 1 out]
        n92 = call "Enum to Array of Enums.vim"("enum"=Hotkey_Type."Macro Hotkey" ("Hotkey Type")) -> ("array of enums"=w235:T1[])
        n93 = Not(x=w246) -> (.not. x?=w243:bool)
        n94 = Sort 1D Array(array=w251) -> (sorted array=w232:T7)
        n95 = Equal?(x=w245, y=w232) -> (x = y?=w244:bool)
        n96 = for {
          tunnel: w235 -> [w256] mode=indexing
          tunnel: w233 -> [w257]
          tunnel: [w256] -> w230 if=w253
          tunnel: w232 -> [w255]
          tunnel: [w253] -> w228
          stop <- w253 stop-if-true
          n97 = case shown="\"Abort Hotkey\"" w256 {
            tunnel: w257 -> [w259 w261]
            tunnel: [w258 w260] -> w254
            frame "Macro Hotkey", Default {
              n98 = Unbundle By Name(w259) -> ("Macro Hotkey"=w258:T7)
            }
            frame "Abort Hotkey" {
              n99 = Unbundle By Name(w261) -> ("Abort Hotkey"=w260:T7)
            }
          }
          n100 = Equal?(x=w254, y=w255) -> (x = y?=w253:bool)
        }
        n101 = Not(x=w228) -> (.not. x?=w227:bool)
        n102 = Format Into String(format string="That key combination is already assigned as the %s.", w230) -> (resulting string=w229:string)  [unwired: 2 in, 1 out]
        n103 = Compound Arithmetic op=AND(w227, w243, w244) -> (w242:bool)
        n104 = call "Already Assigned"("Enable"=w228, "Message"=w229) -> ()  [unwired: 8 in, 2 out]
        n105 = Select(t="Timer: Poll", s=w242, f="Timer: Reset\nUI: Listen") -> (s? t:f=w236:string)
        n106 = call "Enqueue Multiple States.vi"("queue in"=w239, "State(s) at Back"=w236) -> ()  [unwired: 13 in, 1 out]
        n107 = Bundle By Name(cluster=w238, "Last"=w232) -> (w237:T6)
      }
      frame "---------- Macro ----------" {
        # "Do not put any code in this frame.\n(It is a separator no-op. You can make a copy of this frame to create a new Macro frame)"
        n108 = call "Enqueue Multiple States.vi"("queue in"=w262) -> ()  [unwired: 14 in, 1 out]
      }
      frame "Macro: Initialize" {
        w265 = "Data: Initialize\nData: Get Hotkeys\nInitialize Core Data\nUI: Initialize\nUI: Front Panel State >> Open"  # Data: Initialize Data: Get Hotkeys Initialize Core Data UI: Initialize UI: Front Panel State >> Open
        # "Initialization Macro\n(This is called once, when the VI starts)"
        n109 = call "Enqueue Multiple States.vi"("State(s) at Front"=w265, "queue in"=w266) -> ()  [unwired: 13 in, 1 out]
      }
      frame "Macro: Exit" {
        # "Exit Macro\n(This is called once, when the VI exits)"
        n110 = Unbundle By Name(w276) -> ("Core.Close Panel on Exit?"=w275:bool)
        n111 = Select(t="UI: Front Panel State >> Close\n", s=w275, f="") -> (s? t:f=w271:string)
        n112 = Concatenate Strings(w271, "Data: Cleanup\nExit") -> (w269:string)
        n113 = call "Enqueue Multiple States.vi"("State(s) at Front"=w269, "queue in"=w272) -> ()  [unwired: 13 in, 1 out]
      }
      frame "---------- Timer ----------" {
        # "Template Separator\n(You can make a copy of, or modify, this frame)"
        n114 = call "Enqueue Multiple States.vi"("queue in"=w278) -> ()  [unwired: 14 in, 1 out]
      }
      frame "Timer: Reset" {
        n115 = call "Timer FGV.vi"("Mode"=FGV_Actions."Write", "error in (no error)"=w284, "Timer Value (s)"=5.0) -> ("error out"=w283:errorcluster)  [unwired: 6 in, 2 out]
      }
      frame "Timer: Poll" {
        n116 = call "Timer FGV.vi"("Mode"=FGV_Actions."Read", "error in (no error)"=w293) -> ("error out"=w292:errorcluster, "Expired?"=w290:bool)  [unwired: 7 in, 1 out]
        n117 = Select(t="Data: Save Hotkey\nData: Get Hotkeys", s=w290, f="UI: Listen") -> (s? t:f=w286:string)
        n118 = call "Enqueue Multiple States.vi"("queue in"=w287, "State(s) at Back"=w286) -> ()  [unwired: 13 in, 1 out]
      }
    }
  }
  n119 = Merge Errors(w9, w8) -> (w10:errorcluster)
  n120 = Release Queue(queue=w11, error in (no error)=w10) -> (error out=→"error out":errorcluster)  [unwired: 1 in, 2 out]
